vi "DefaultPersonality_5745_FPGA.vi"() -> ()   [LabVIEW 2021, in "GettingStarted_5745_FPGA.lvlib"]
uses:
  GettingStarted_5745_FPGA.lvlib
  <instrlib>/_niInstr/Streaming/v1/Common/Stream State.ctl
  <vilib>/Platform/TimedLoop/XDataNode/timing_clust.ctl
  <vilib>/Platform/TimedLoop/XDataNode/nitl_modes.ctl
  <vilib>/Platform/TimedLoop/XDataNode/wakeup.ctl
  <instrlib>/FlexRIO/API/FPGA/v1/Types/Start Trigger IO Resources.ctl
  <vilib>/rvi/Emulation/niFpgaSctlEmulationGetInTimedLoop.vi
  <vilib>/rvi/Emulation/niFpgaEmulationReportErrorSimple.vi
  <vilib>/rvi/Emulation/niFpgaGetClockAttributes.vi
  <vilib>/rvi/Emulation/niFpgaCriticalErrorInLSC.vi
  <vilib>/rvi/eio/common/nirviEmuTemplateMethod_errors.vi
  <vilib>/rvi/DataTransferAndStorage/Container/Common/niFpgaContainerGetUniqueNameForEmu.vi
  <vilib>/rvi/DataTransferAndStorage/Container/Common/niFpgaContainerSetEmuInfo.vi
  <vilib>/rvi/eio/common/nirviEmuReportErrorAndStop.vi
  <vilib>/rvi/interface/RandomDataEmulation/nirviRandomDataMultiElementFPGAFIFO.vi
  <instcachedir>/0/nirviRandomDataMultiElementFPGAFIFO_3E9965BA1FAD4E7B8DABA31768A09B1F.lvgen/nirviRandomDataMultiElementFPGAFIFO_3E9965BA1FAD4E7B8DABA31768A09B1F_001.vi
  <vilib>/rvi/interface/RandomDataEmulation/niFpgaRandomDataHandleErrors.vi
  <vilib>/rvi/DataTransferAndStorage/Container/Common/niFpgaContainerExecOnDevCompGetState.vi
  <vilib>/rvi/Emulation/niFpgaEmulationIsFPGAContextNoSignature.vi
  <vilib>/rvi/errors/niFpgaSetErrorForExecOnDevCompSimple.vi
  <vilib>/rvi/FIFO/Fifo_Resource/nirvififoEmulationSetSize.vi
  <vilib>/rvi/FIFO/Fifo_Resource/nirviFifoEmulationQueueMgr.vi
  <instcachedir>/0/nirviFifoEmulationQueueMgr_E5CAEC123FF24DC58D834DCA3CDAA9B5.lvgen/nirviFifoEmulationQueueMgr_E5CAEC123FF24DC58D834DCA3CDAA9B5_008.vi
  <vilib>/rvi/FIFO/Fifo_Resource/nirvififoEmulationDetermineInputValidOut.vi
  <vilib>/rvi/FIFO/Fifo_Resource/nirvififoEmulationCreateLock.vi
  <vilib>/rvi/Emulation/niFpgaProcessEmulError.vi
  <vilib>/rvi/FIFO/Fifo_Resource/nirvififoEmulationObtainLock.vi
  <vilib>/rvi/FIFO/Fifo_Resource/nirvififoEmulationReleaseLock.vi
  <vilib>/rvi/occurrence/nirviWaitOnOccurrenceBase.vi
  <vilib>/rvi/errors/nirviReportUnexpectedCaseInternalError.vi
  <vilib>/rvi/errors/nirviReportUnexpectedCaseInternalError (U32).vi
  <vilib>/Utility/error.llb/Clear Errors.vi
  7192f61d-e408-4cca-baff-cb10c33219c0.vi
  <vilib>/Platform/TimedLoop/XDataNode/XDataNode.xnode
  <vilib>/eio/EIONode/EIONode.xnode
  <vilib>/rvi/LocalResourceManager/LocalResourceManager.xnode
  <vilib>/rvi/DataTransferAndStorage/Container/XNode/niFpgaContainer.xnode
  <vilib>/rvi/interface/RandomDataEmulation/nirviRandomDataFpgaMultiElementTemplate.vi
  <vilib>/rvi/FIFO/Fifo_Resource/niFpgaFifoEmulationRefIn.vi
  <vilib>/Platform/TimedLoop/XDataNode/XDNodeRunTimeDep.lvlib
  <instrlib>/_niInstr/Streaming/v1/FPGA/niInstr Streaming v1 FPGA.lvlib
  <instrlib>/FlexRIO/API/FPGA/v1/FlexRIO API FPGA v1.lvlib
  <instrlib>/FlexRIO/API/FPGA/v1/IO/NI5745/FlexRIO 5745 FPGA v1.lvlib
  <instrlib>/_niInstr/Streaming/v1/Common/niInstr Streaming v1 Common.lvlib
panel:
  in  "User-defined Start Trigger - AO":bool
  in  "flexrio.trigger.start.cfg 0":u16
  out "written elements":u64
  out "buffer size in elements":u64
  out "IO Socket\\AO Ready For Input":bool
  in  "stream.request state 0":T1
  in  "stream.num samples 0":u64
  out "stream.metadata 0":u64
  out "stream.samples transferred 0":u64
  out "stream.state 0":T1
  in  "reset circular buffer":bool
  out "flexrio.module.io ready 0":bool
  out "flexrio.module.io error 0":i32
  # "Device Utilization\n---------------------------\nTotal Slices: 38.6% (11706 out of 30300)\nSlice Registers: 13.0% (62879 out of 484800)\nSlice LUTs: 22.7% (54915 out of 242400)\nBlock RAMs: 27.5% (165 out of 600)\nDSP48s: 0.0% (0 out of 1920))\n\nNote: Utilization numbers are for the KU040. Exact values will vary for the KU060 and KU035."
  # "AO Stream Configuration"
  # "Module Status"
  # "AO Buffer Configuration"
  # "User-defined Controls"
  # "AO Trigger Configuration"
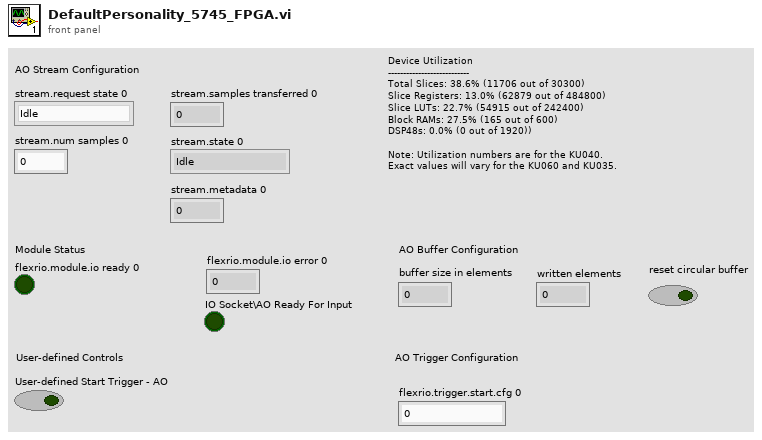
[diagram p1: front panel]
types:
  T1 = typedef "niInstr Streaming v1 Common.lvlib/Stream State.ctl" = enum8{"Idle", "Finite Transfer", "Continuous", "Done", "Error", "Not Ready", "Cancel"}
  T2 = typedef "XDNodeRunTimeDep.lvlib/timing_clust.ctl" = cluster{"Expected End [f-1]":u64, "Actual End [f-1]":u64, "Finished Late? [f-1]":bool, "Expected End [i-1]":u64, "Actual End [i-1]":u64, "Finished Late? [i-1]":bool, "Expected Start [i]":u64, "Actual Start [i]":u64, "Expected Start [f]":u64, "Actual Start [f]":u64, "Source Name":string, "Structure Name":string, "Period":i64, "Deadline":i64, "Offset":i64, "Start":i64, "Priority":i32, "Timeout":i32, "Mode":T3, "Wakeup Reason":T4, "Error":errorcluster, "Source Type":string, "Secondary Source Type":string, "Global End Time":u64, "Global Start Time":u64, "Frame Duration":u64, "Iteration Duration":u64, "Assigned CPU":i32, "I/O Scan Engine Mode":u32}
  T3 = typedef "XDNodeRunTimeDep.lvlib/nitl_modes.ctl" = enum32{"No Change", "Process missed periods, maintain original phase", "Discard missed periods, maintain original phase", "Process missed periods, ignore original phase", "Discard missed periods, ignore original phase"}
  T4 = typedef "XDNodeRunTimeDep.lvlib/wakeup.ctl" = enum32{"Normal", "Aborted", "Asynchronous wakeup", "Timing source error", "Timed loop error", "Timeout"}
  T5 = typedef "FlexRIO API FPGA v1.lvlib/Start Trigger IO Resources.ctl" = cluster{"start trigger":refnum<k21>, "started event":refnum<k21>, "start trigger for export":refnum<k21>, "start trigger for tclk":refnum<k21>}
  T6 = typedef "FlexRIO API FPGA v1.lvlib/Start Trigger Control.ctl" = cluster{"arm start":bool, "done":bool}
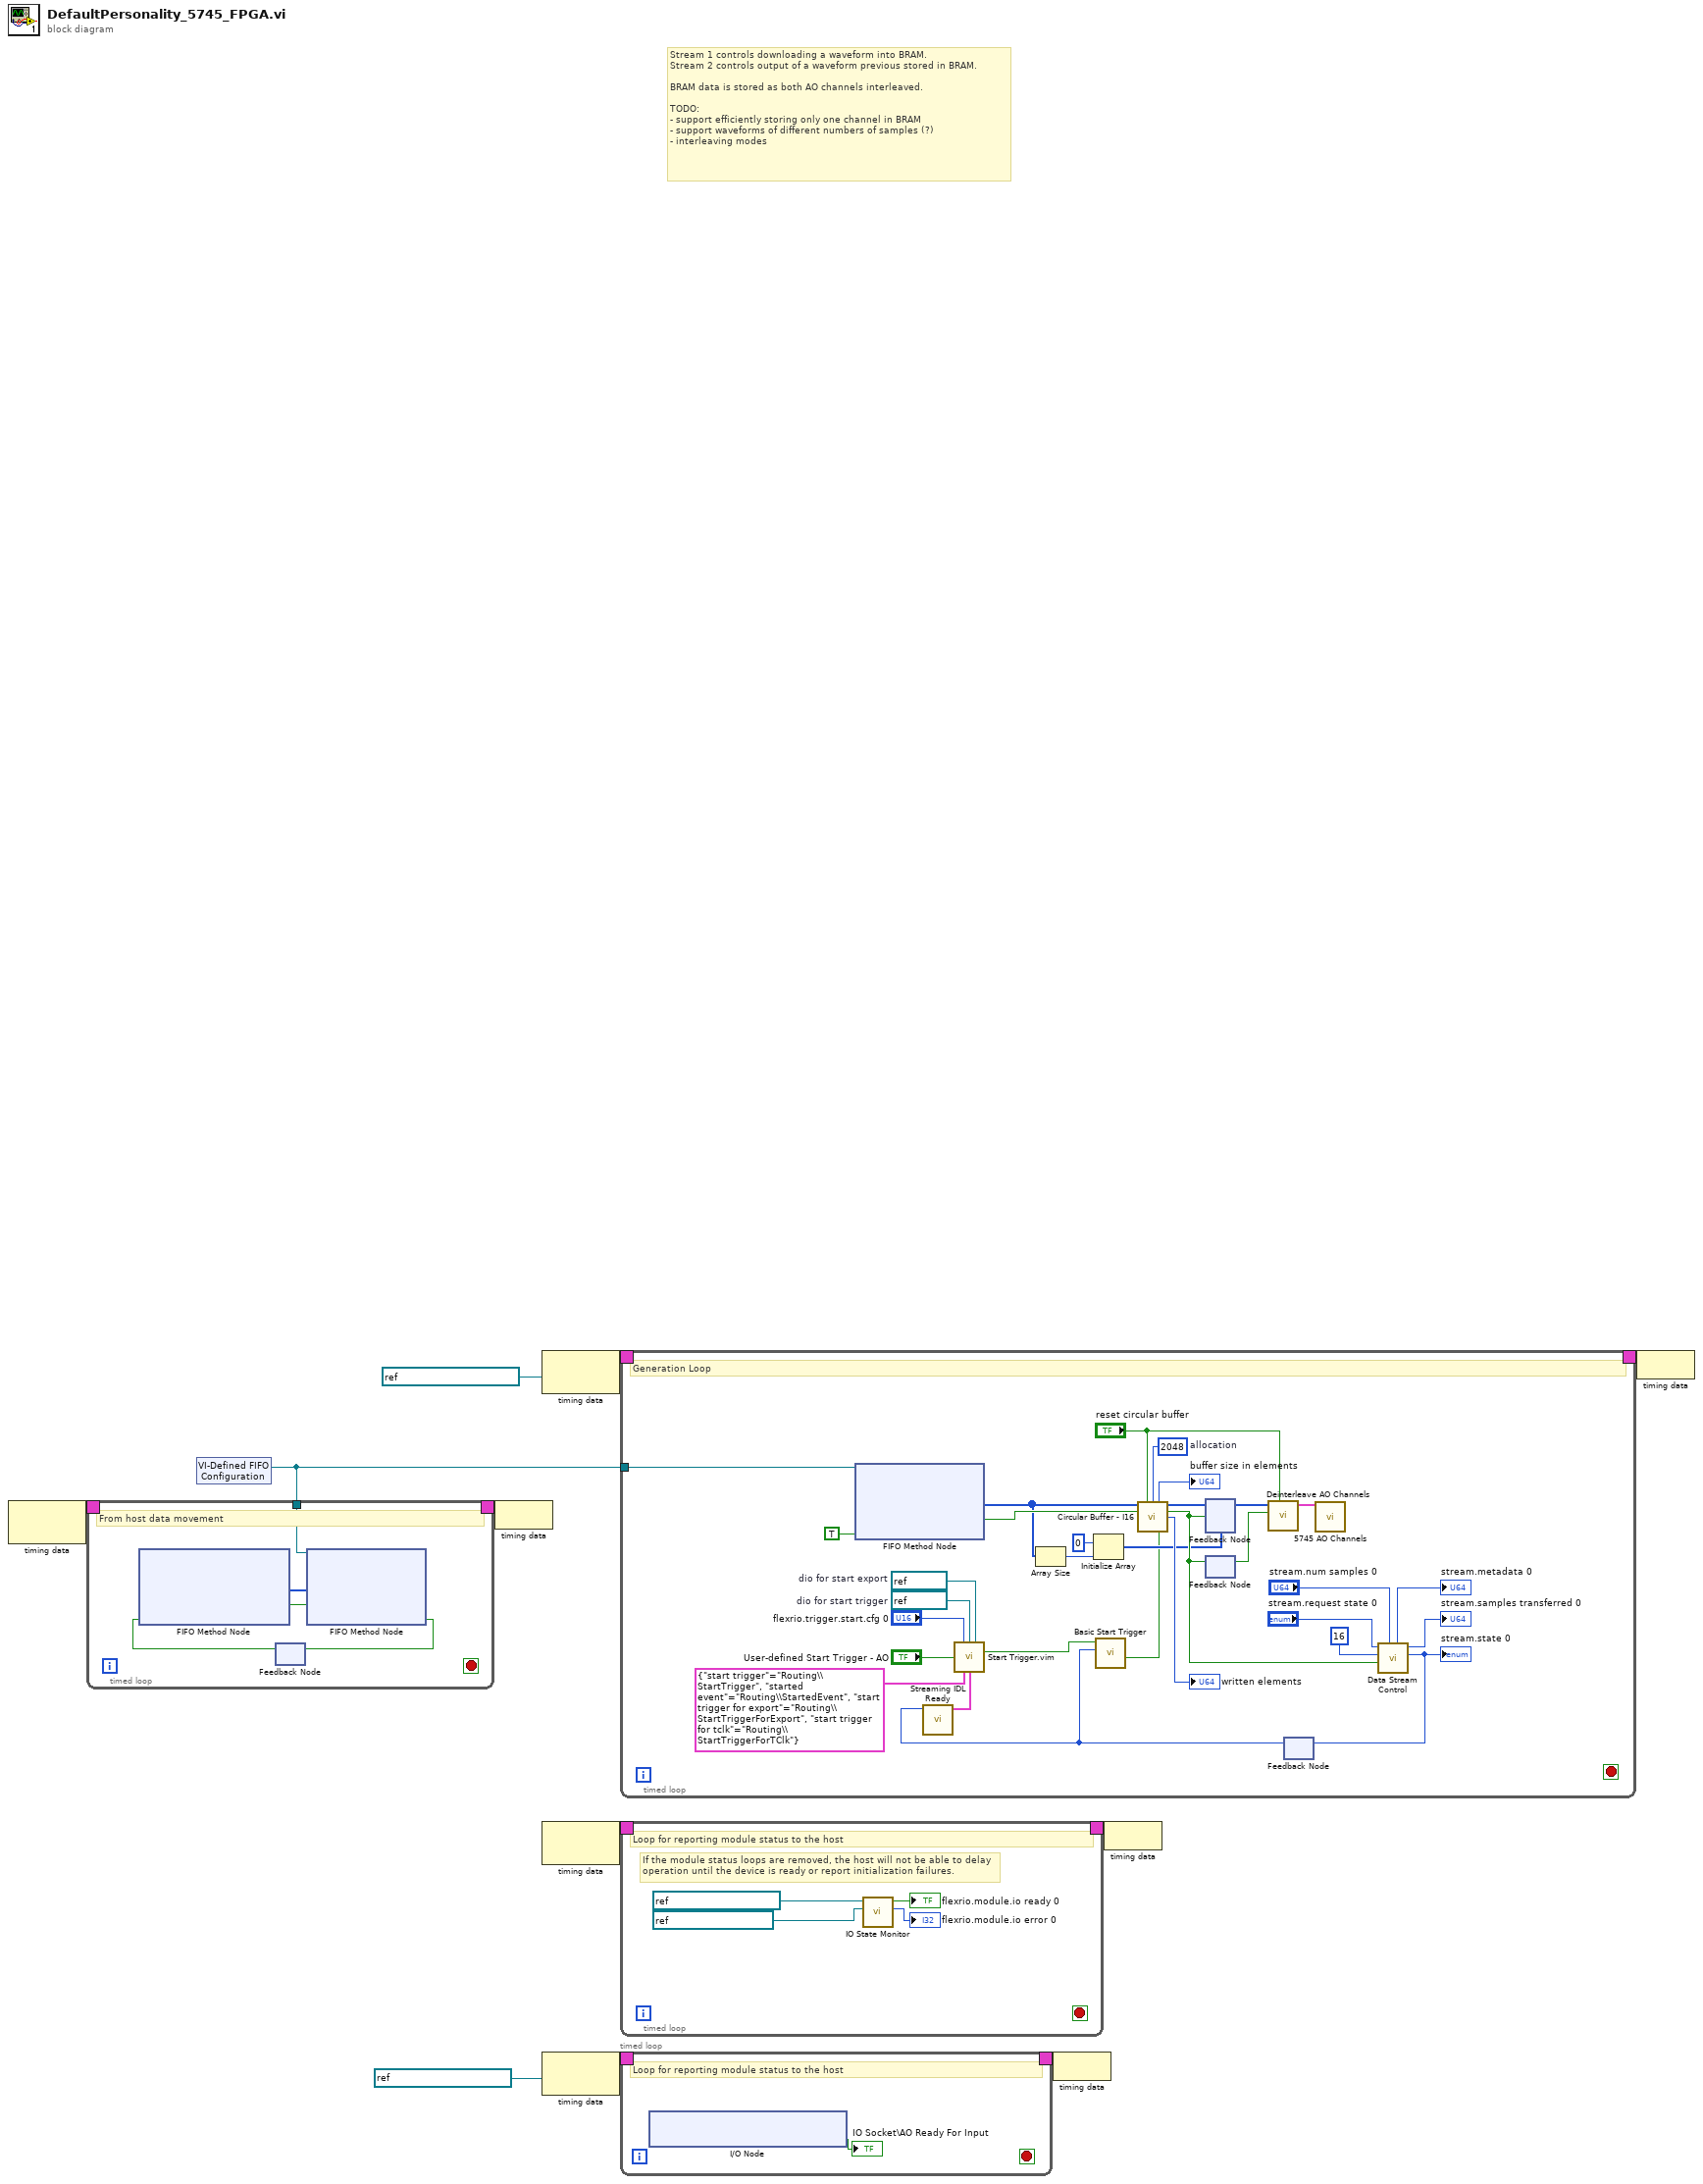
[diagram p0: block diagram]
diagram:
  # "Stream 1 controls downloading a waveform into BRAM.\nStream 2 controls output of a waveform previous stored in BRAM.\n\nBRAM data is stored as both AO channels interleaved.\n\nTODO:\n- support efficiently storing only one channel in BRAM\n- support waveforms of different numbers of samples (?)\n- interleaving modes"
  n1 = node-c288() -> (w3:T2)  [unwired: 1 in]
  n2 = xnode "VI-Defined FIFO Configuration"() -> ("FIFO Out"=w1:refnum<k21>)
  n3 = timed-loop {
    timing: w3 -> [_]
    timing-out: [_] -> w2
    tunnel: w1 -> [w12]
    stop <- _ stop-if-true
    # "From host data movement"
    n4 = feedback #1() -> (w16:bool)  [unwired: 1 in]
    n5 = xnode ("FIFO Method Node")("Ready for Output"=w16) -> ("Element"=w13:i16[], "Output Valid"=w14:bool)  [unwired: 1 in, 1 out]
    n6 = xnode ("FIFO Method Node")("Element"=w13, "Input Valid"=w14, "FIFO In"=w12) -> ("Ready for Input"=w15:bool)  [unwired: 1 out]
    n7 = feedback-in #1(w15) -> ()
  }
  n8 = node-c288(w2) -> ()
  n9 = node-c288(refnum<k21> "IO Socket\\Data Clock" ("Source Name")) -> (w11:T2)
  n10 = node-c288() -> (w8:T2)  [unwired: 1 in]
  n11 = node-c288(refnum<k21> "IO Socket\\Data Clock" ("Source Name")) -> (w6:T2)
  n12 = timed-loop {
    timing: w11 -> [_]
    timing-out: [_] -> w10
    tunnel: w1 -> [w28]
    stop <- _ stop-if-true
    w23 = refnum<k21> "DIO 0"  # dio for start trigger
    w22 = refnum<k21> "DIO 1"  # dio for start export
    w34 = 2048  # allocation
    # "Generation Loop"
    n13 = xnode ("FIFO Method Node")("Ready for Output"=TRUE, "FIFO In"=w28) -> ("Element"=w36:i16[], "Output Valid"=w41:bool)  [unwired: 1 out]
    n14 = Array Size(array=w36) -> (size(s)=w43:i32)
    n15 = Initialize Array(0 ("element"), w43) -> (w38:i32[])
    n16 = feedback #2(w38) -> (w44:i32[])
    n17 = feedback #3() -> (w47:bool)  [unwired: 1 in]
    n18 = call "Deinterleave AO Channels.vi"("clear"="reset circular buffer", "data valid"=w47, "interleaved data"=w44) -> ("channel array"=w45:cluster{fxp<+/-,12,1>[]}[])  [unwired: 8 in]
    n19 = feedback #4() -> (w20:T1)  [unwired: 1 in]
    n20 = call <instrlib>:"Streaming IDL Ready.vi"("stream.state"=w20) -> ("start trigger control"=w25:T6)  [unwired: 10 in]
    n21 = call "Start Trigger.vim"("flexrio.trigger.start.cfg 0"="flexrio.trigger.start.cfg 0", "dio start"=w23, "dio for start export"=w22, "user-defined start trigger"="User-defined Start Trigger - AO", "trigger io resources"=T5 {"start trigger"="Routing\\StartTrigger", "started event"="Routing\\StartedEvent", "start trigger for export"="Routing\\StartTriggerForExport", "start trigger for tclk"="Routing\\StartTriggerForTClk"}, "start trigger control"=w25) -> ("conditioned start trigger"=w24:bool)  [unwired: 7 in, 2 out]
    n22 = call <instrlib>:"Basic Start Trigger.vi"("stream.state"=w20, "start trigger"=w24) -> ("data valid"=w29:bool)  [unwired: 9 in]
    n23 = call <instrlib>:"Circular Buffer - I16.vi"("write data"=w36, "reset"="reset circular buffer", "allocation (clock cycles)"=w34, "write data valid"=w41, "ready for output"=w29) -> ("buffer size in elements"=→"buffer size in elements":u64, "read data"=w35:i16[], "read data valid"=w48:bool, "written elements"=→"written elements":u64)  [unwired: 7 in]
    n24 = feedback-in #2(w35, w48) -> ()
    n25 = feedback-in #3(w48) -> ()
    n26 = call <instrlib>:"5745 AO Channels.vi"("all channels"=w45) -> ()  [unwired: 15 in]
    n27 = call <instrlib>:"Data Stream Control.vi"("stream.num samples 0"="stream.num samples 0", "data valid"=w48, "element count"=u16 16, "stream.request state 0"="stream.request state 0") -> ("stream.state 0"=w27:T1, "stream.samples transferred 0"=→"stream.samples transferred 0":u64, "stream.metadata 0"=→"stream.metadata 0":u64)  [unwired: 3 in, 2 out]
    "stream.state 0" <- w27
    n28 = feedback-in #4(w27) -> ()
  }
  n29 = timed-loop {
    timing: w8 -> [_]
    timing-out: [_] -> w7
    stop <- _ stop-if-true
    # "If the module status loops are removed, the host will not be able to delay operation until the device is ready or report initialization failures."
    # "Loop for reporting module status to the host"
    n30 = call <instrlib>:"IO State Monitor.vi"("io error resource"=refnum<k21> "IO Socket\\IO Error" ("FPGA I/O In"), "io ready resource"=refnum<k21> "IO Socket\\IO Ready" ("FPGA I/O In")) -> ("flexrio.module.io error 0"=→"flexrio.module.io error 0":i32, "flexrio.module.io ready 0"=→"flexrio.module.io ready 0":bool)  [unwired: 8 in]
  }
  n31 = timed-loop {
    timing: w6 -> [_]
    timing-out: [_] -> w5
    stop <- _ stop-if-true
    # "Loop for reporting module status to the host"
    n32 = xnode "I/O Node"() -> ("IO Socket\\AO Ready For Input"=→"IO Socket\\AO Ready For Input":bool)  [unwired: 1 in, 1 out]
  }
  n33 = node-c288(w5) -> ()
  n34 = node-c288(w7) -> ()
  n35 = node-c288(w10) -> ()
